vi "Get Array Targets.vi"(7 "Load Stored Targets?(T)":bool=TRUE, 8 "error in (no error)":errorcluster, 11 "Dependency Sources":refnum<class "Dependency Source.lvclass">[](array[class])) -> (0 "error out":errorcluster, 1 "All Success?":bool, 2 "External Targets":T3[](array[typedef]), 3 "Internal Targets":T2[](array[typedef]), 4 "Unhandled Targets":T1[](array[typedef]), 5 "Success? Array":bool[](array[boolean]))   [LabVIEW 2019, in "Project.Dependencies Finder.lvlib" / "Dependency Source.lvclass"]
doc: "Get internal and external targets for an array of dependency sources."
uses:
  Dependency Source.lvclass
  Ctl/Ctl_External Target Element.ctl
  Ctl/Ctl_Internal Target Element.ctl
  Ctl/Ctl_Dependency Element.ctl
  Project.Dependencies Finder.lvlib
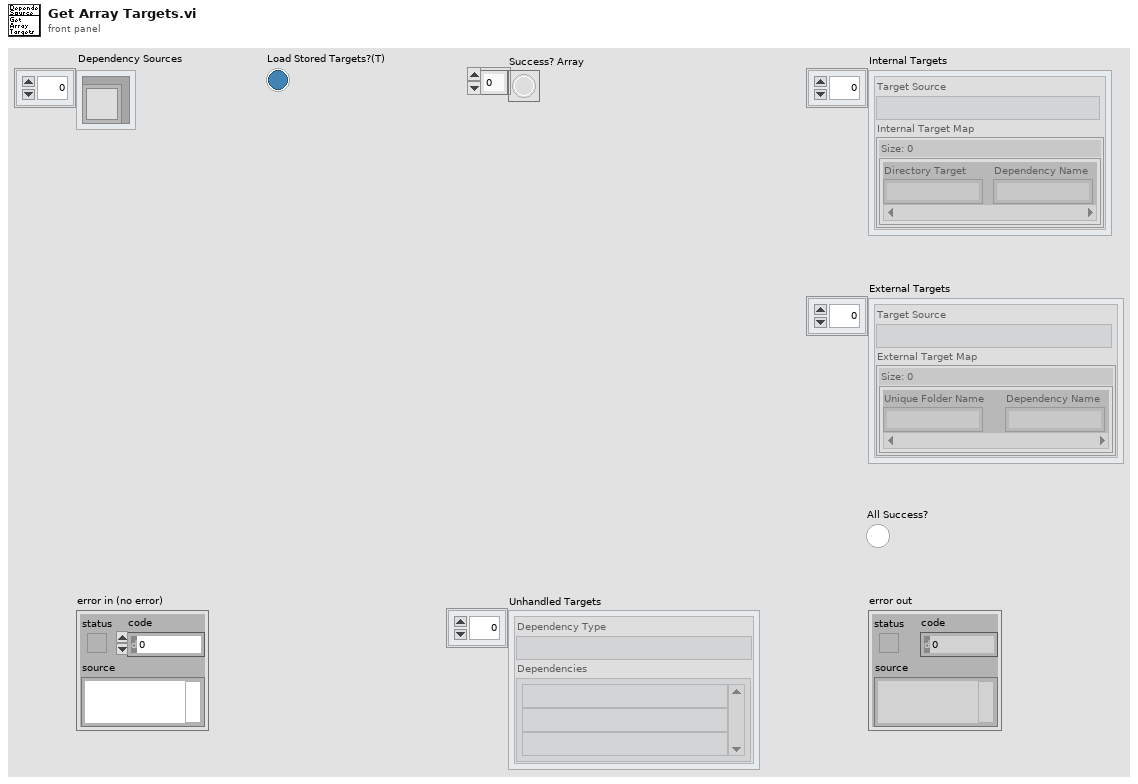
[diagram p1: front panel]
types:
  T1 = typedef "Project.Dependencies Finder.lvlib/Ctl_Dependency Element.ctl" = cluster{"Dependency Type":string, "Dependencies":string[]}
  T2 = typedef "Project.Dependencies Finder.lvlib/Ctl_Internal Target Element.ctl" = cluster{"Target Source":string, "Internal Target Map":map{string, string}}
  T3 = typedef "Project.Dependencies Finder.lvlib/Ctl_External Target Element.ctl" = cluster{"Target Source":string, "External Target Map":map{string, string}}
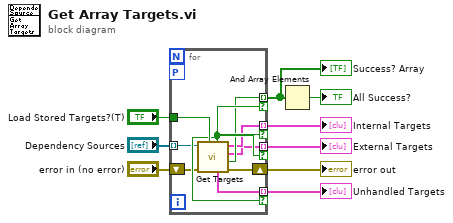
[diagram p0: block diagram]
diagram:
  n1 = for {
    tunnel: [w14] -> w7 mode=indexing if=w17
    tunnel: [w13] -> w6 mode=indexing if=w17
    tunnel: [w12] -> w5 mode=indexing if=w17
    tunnel: "Dependency Sources" -> [w11] mode=indexing
    shift-right: [w16] -> w9
    shift-left: "error in (no error)" -> [w10]
    workers-P: _ -> [_]
    tunnel: [w15] -> w2 mode=indexing if=w17
    tunnel: "Load Stored Targets?(T)" -> [w18]
    n2 = call "Get Targets.vi"("Load Stored Targets?(T)"=w18, "error in (no error)"=w10, "Dependency Source in"=w11) -> ("error out"=w16:errorcluster, "Success?"=w14:bool, "External Targets"=w12:T3, "Internal Targets"=w13:T2, "Unhandled Targets"=w15:T1, "Valid Dependency Source?"=w17:bool)  [unwired: 3 in]
  }
  "error out" <- w9
  "Internal Targets" <- w6
  "External Targets" <- w5
  "Success? Array" <- w7
  "Unhandled Targets" <- w2
  n3 = And Array Elements(Boolean array=w7) -> (logical AND=→"All Success?":bool)
